vi "TDMS_File_Constants Globals.vi"() -> ()   [LabVIEW 2019]
uses:
  TDMS Constants.ctl
panel:
  out "PowGrp0":T1={"Channel Names"=["", "", "", "", "", "", "", "", "", "", "", ""], "Channel Units"=["", "", "", "", "", "", "", "", "", "", "", ""], "TDMS File Suffix"="PowGrp0", "Channel Datatype"=["", "", "", "", "", "", "", "", "", "", "", ""]}
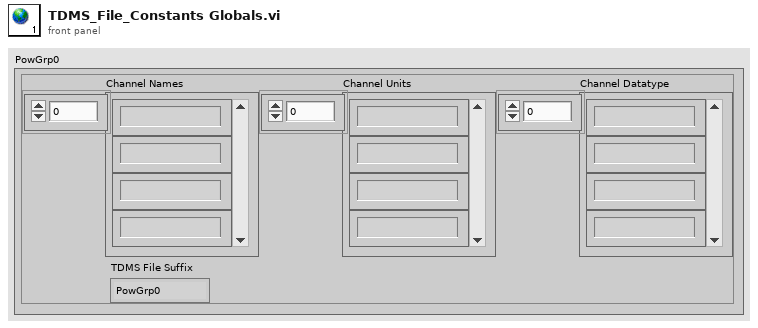
[diagram p1: front panel]
types:
  T1 = typedef "TDMS Constants.ctl" = cluster{"Channel Names":string[], "Channel Units":string[], "TDMS File Suffix":string, "Channel Datatype":string[]}
diagram:
